vi "Parseval's Theorem.vi"() -> ()   [LabVIEW 2023]
doc: "This example demonstrates the discrete-time version of Parseval's relation which in simple terms states that the total energy in a signal is the same in both time and frequency domains."
uses:
  <vilib>/Analysis/2dsp.llb/Real FFT.vi
  <vilib>/Analysis/NI_AALPro.lvlib
  <vilib>/Analysis/NI_AALBase.lvlib
panel:
  out "Fourier Transform":dbl[](graph)
  out "Waveform Graph":dbl[](graph)
  out "1/N Sum[|X(k)|^2]":dbl=1528.6213257631189 format="%0.4f"
  out "Sum[x(n) x(n)]":dbl=1528.621325763123 format="%0.4f"
  # "Overview: This example demonstrates the discrete-time version of Parseval's relation which states that the total energy in a signal is the same in both the time and frequency domains. \nRequirements: LabVIEW Full Development System\nInstructions:\n1. Run the VI.\n2. Verify that the Time Domain and Frequency Domain energy values are equal."
  # "Frequency Domain"
  # "Time Domain"
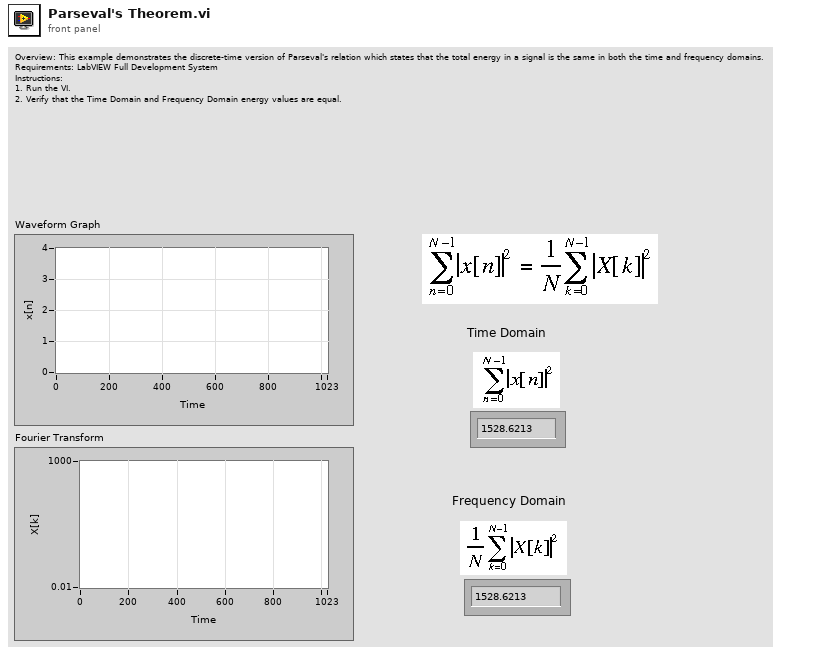
[diagram p1: front panel]
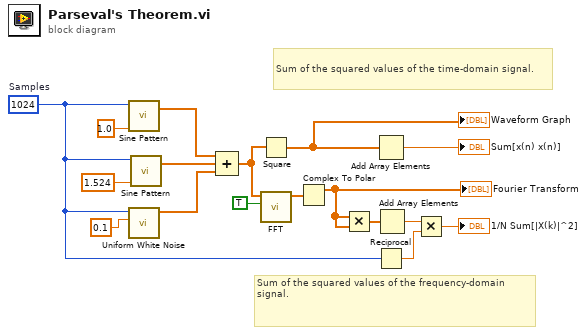
[diagram p0: block diagram]
diagram:
  w3 = 1024  # Samples
  # "Sum of the squared values of the frequency-domain signal."
  # "Sum of the squared values of the time-domain signal."
  n1 = call <vilib>:"Sine Pattern.vi"("cycles"=1.0, "samples"=w3) -> ("Sinusoidal Pattern"=w12:dbl[])  [unwired: 2 in, 1 out]
  n2 = call <vilib>:"Uniform White Noise.vi"("amplitude"=0.1, "samples"=w3) -> ("uniform white noise"=w1:dbl[])  [unwired: 8 in, 1 out]
  n3 = call <vilib>:"Sine Pattern.vi"("cycles"=1.524, "samples"=w3) -> ("Sinusoidal Pattern"=w2:dbl[])  [unwired: 2 in, 1 out]
  n4 = Compound Arithmetic op=ADD(w12, w2, w1) -> (w6:dbl[])
  n5 = Square(x=w6) -> (x^2=w10:dbl[])
  "Waveform Graph" <- w10
  n6 = call-poly <vilib>:"FFT.vi"("shift?"=TRUE, "X"=w6) -> ("FFT {X}"=w14:cdb[])  [unwired: 8 in, 1 out]
  n7 = Complex To Polar(r * e^(i*theta)=w14) -> (r=w7:dbl[])  [unwired: 1 out]
  "Fourier Transform" <- w7
  n8 = Multiply(x=w7, y=w7) -> (x*y=w8:dbl[])
  n9 = Add Array Elements(numeric array=w10) -> (sum=→"Sum[x(n) x(n)]":dbl)
  n10 = Reciprocal(x=w3) -> (1/x=w13:dbl)
  n11 = Add Array Elements(numeric array=w8) -> (sum=w16:dbl)
  n12 = Multiply(x=w16, y=w13) -> (x*y=→"1/N Sum[|X(k)|^2]":dbl)
